vi "OCR_Seperate characters into bit arrays.vi"(7 "Color Set":T2={"BG"=255, "FG"=16711680}, 8 "Error":errorcluster, 9 "Column Type Array":T3[](array[typedef]), 11 "2D Image":u32[][](array[colorbox])) -> (0 "Error Out":errorcluster, 2 "All Good Out":bool, 3 "Char Array Out":T1[](array[typedef]))   [LabVIEW 2009]
doc: "Builds the bit character array from Image, color set, and column type array"
uses:
  Controls/Enum/ENUM_Line Letter Type.ctl
  Controls/Cluster/Cluster_Text Color Set.ctl
  Controls/String_Picture/String Char Normal.ctl
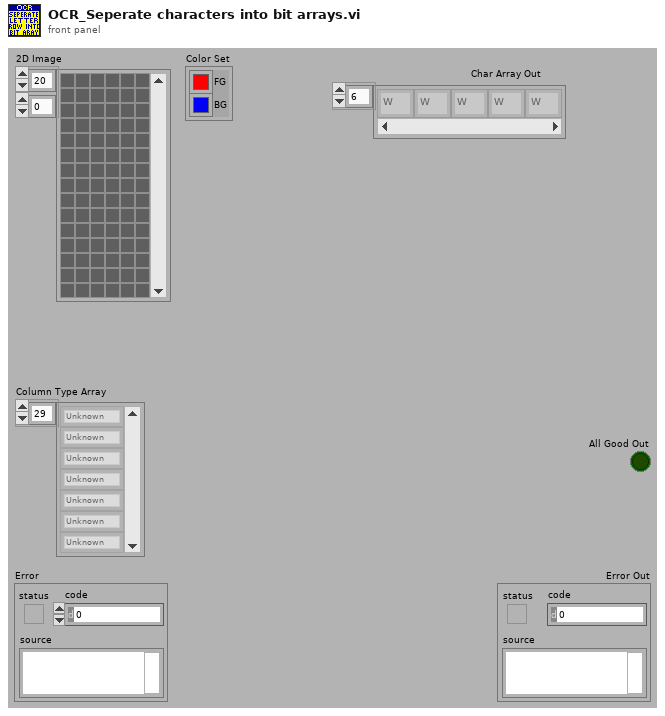
[diagram p1: front panel]
types:
  T1 = typedef "String Char Normal.ctl" = string
  T2 = typedef "Cluster_Text Color Set.ctl" = cluster{"BG":u32, "FG":u32}
  T3 = typedef "ENUM_Line Letter Type.ctl" = enum16{"Unknown", "Letter", "Seperator", "Seperator or Letter"}
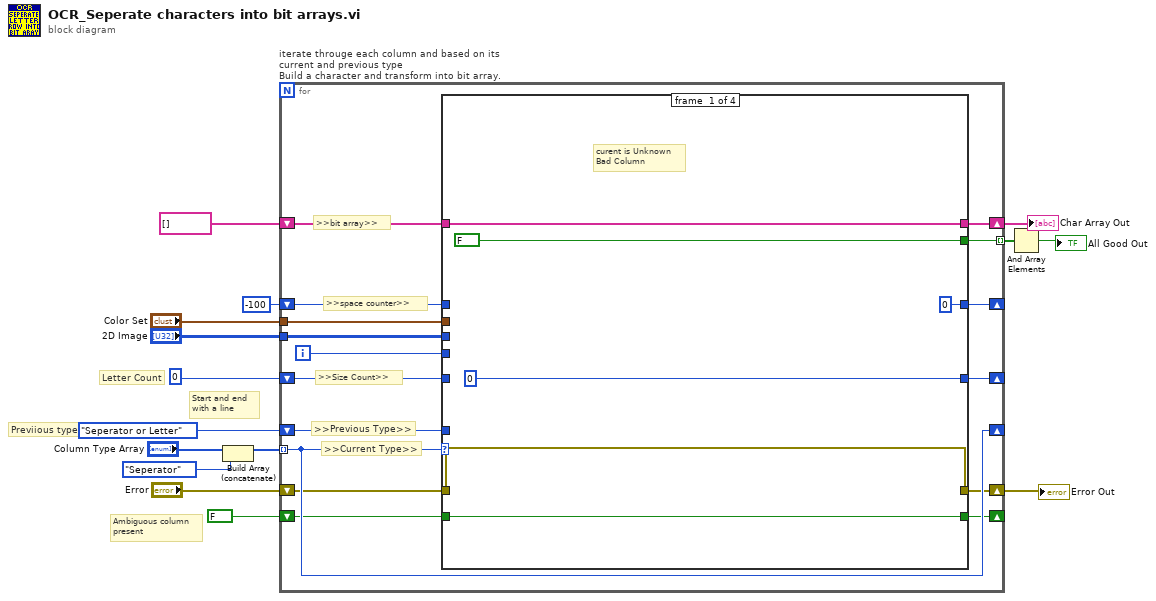
[diagram p0: block diagram]
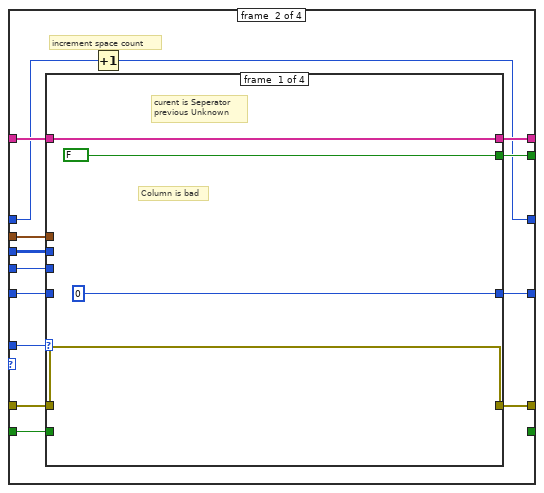
[diagram p2: hidden frame]
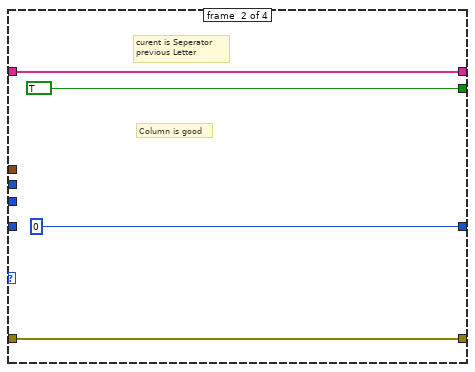
[diagram p3: hidden frame]
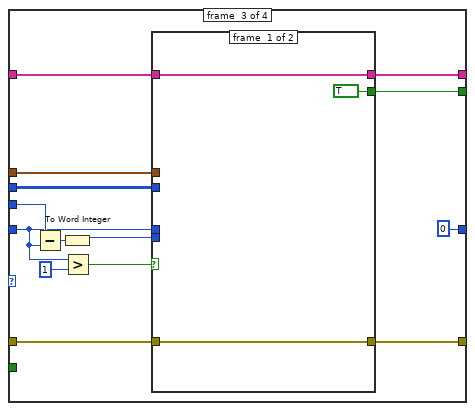
[diagram p4: hidden frame]
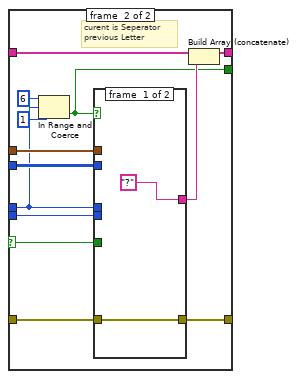
[diagram p5: hidden frame]
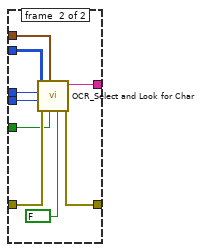
[diagram p6: hidden frame]
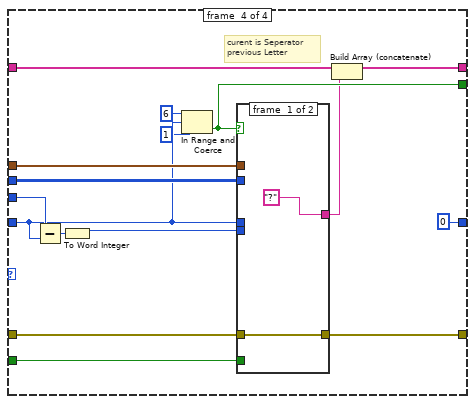
[diagram p7: hidden frame]
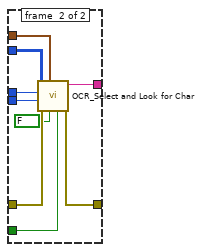
[diagram p8: hidden frame]
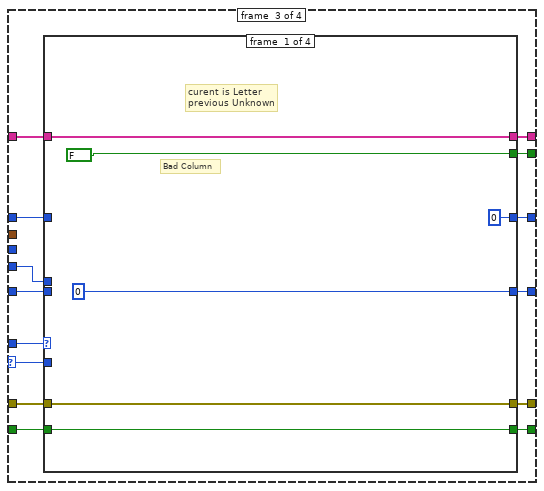
[diagram p9: hidden frame]
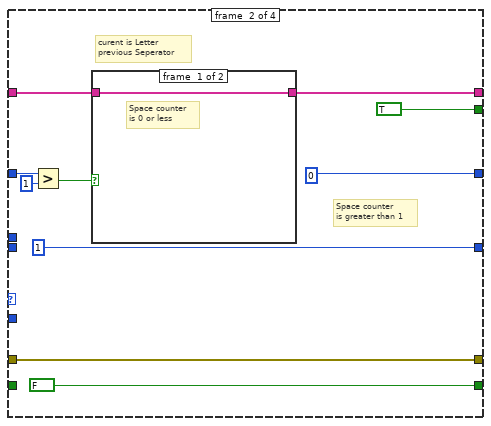
[diagram p10: hidden frame]
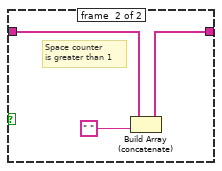
[diagram p11: hidden frame]
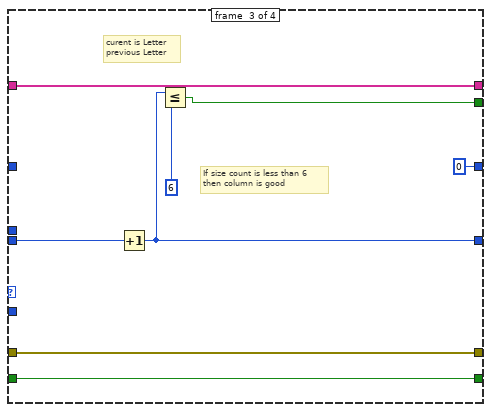
[diagram p12: hidden frame]
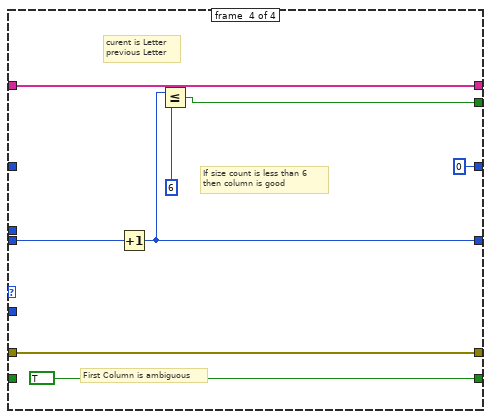
[diagram p13: hidden frame]
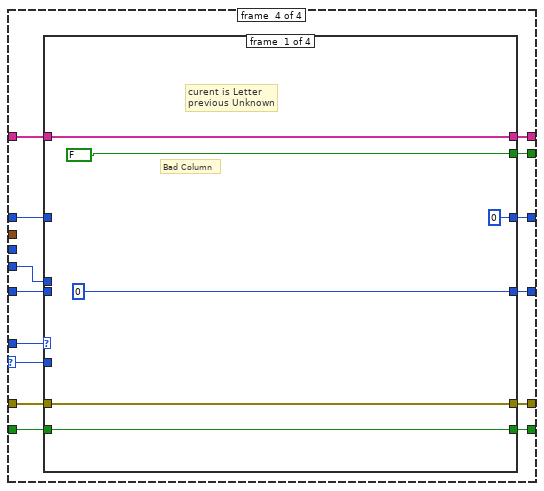
[diagram p14: hidden frame]
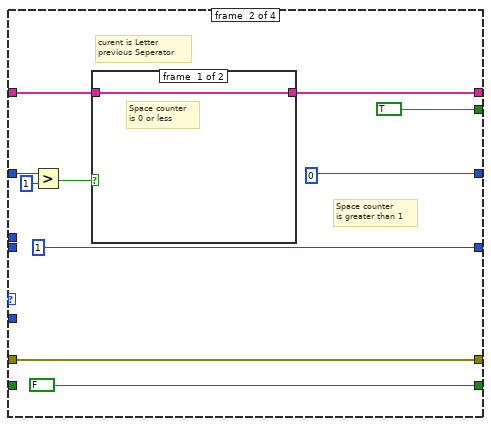
[diagram p15: hidden frame]
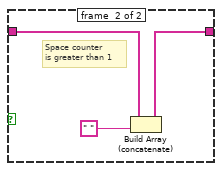
[diagram p16: hidden frame]
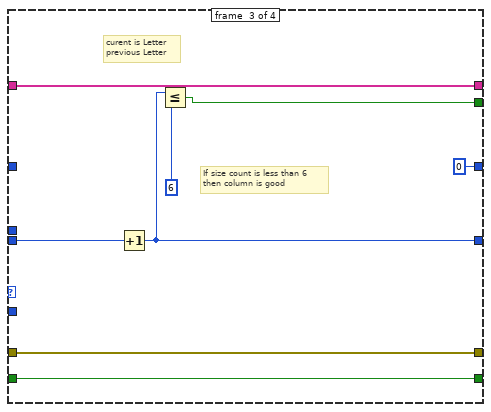
[diagram p17: hidden frame]
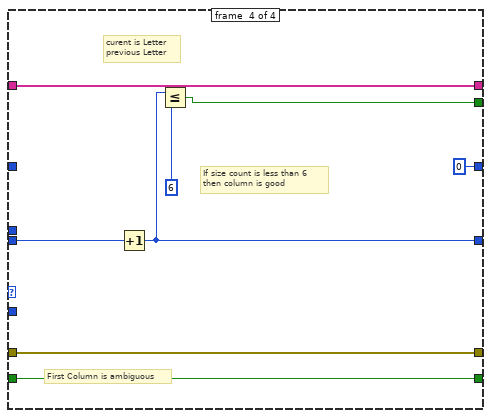
[diagram p18: hidden frame]
diagram:
  # "Ambiguous column\npresent"
  # "Start and end\nwith a line"
  # "Previious type"
  # "Letter Count"
  n1 = Build Array (concatenate)("Column Type Array", ENUM_Line_Letter_Type."Seperator" ("Type Out")) -> (w11:T3[])
  n2 = for "iterate througe each column and based on its current and previous type\nBuild a character and transform into bit array." {
    tunnel: w11 -> [w27] mode=indexing
    shift-right: [w18] -> w14
    shift-left: "Error" -> [w19]
    shift-right: [w29] -> _
    shift-left: 0 -> [w30]
    shift-right: [w27] -> _
    shift-left: ENUM_Line_Letter_Type."Seperator or Letter" ("Type Out") -> [w31]
    tunnel: "2D Image" -> [w26]
    shift-right: [w25] -> w5
    shift-left: T1[] [] ("Bit Char Array Out") -> [w24]
    tunnel: "Color Set" -> [w23]
    tunnel: [w22] -> w9 mode=indexing
    shift-right: [w20] -> _
    shift-left: -100 -> [w21]
    shift-right: [w16] -> _
    shift-left: FALSE -> [w17]
    i -> [w28]
    # ">>Size Count>>"
    # ">>Previous Type>>"
    # ">>Current Type>>"
    # ">>bit array>>"
    # ">>space counter>>"
    n3 = case shown="\"Seperator\"" w27 {
      selector: w27 -> [_ _ w132 w182]
      tunnel: w31 -> [_ w48 w138 w188]
      tunnel: w30 -> [_ w50 w140 w190]
      tunnel: [0 w51 w141 w191] -> w29
      tunnel: w28 -> [_ w49 w139 w189]
      tunnel: w26 -> [_ w47 _ _]
      tunnel: [w36 w46 w136 w186] -> w25
      tunnel: w24 -> [w36 w45 w137 w187]
      tunnel: w23 -> [_ w44 _ _]
      tunnel: [FALSE w43 w135 w185] -> w22
      tunnel: w21 -> [_ w42 w134 w184]
      tunnel: [0 w41 w133 w183] -> w20
      tunnel: w19 -> [w33 w40 w129 w179]
      tunnel: [w33 w39 w128 w178] -> w18
      tunnel: w17 -> [w32 w38 w130 w180]
      tunnel: [w32 _ w131 w181] -> w16
      frame #0 {
        # "curent is Unknown\nBad Column"
      }
      frame #1 {
        # "increment space count"
        n4 = case shown="\"Letter\"" w48 {
          tunnel: [0 0 0 0] -> w51
          tunnel: w50 -> [_ _ w62 w104]
          tunnel: w49 -> [_ _ w66 w109]
          tunnel: w47 -> [_ _ w68 w111]
          tunnel: [w54 w58 w71 w114] -> w46
          tunnel: w45 -> [w54 w58 w70 w113]
          tunnel: w44 -> [_ _ w69 w112]
          tunnel: [FALSE TRUE w63 w106] -> w43
          tunnel: w40 -> [w52 w56 w67 w110]
          tunnel: [w52 w56 w64 w107] -> w39
          tunnel: w38 -> [_ _ _ w105]
          frame #0 {
            # "curent is Seperator\nprevious Unknown"
            # "Column is bad"
          }
          frame #1 {
            # "Column is good"
            # "curent is Seperator\nprevious Letter"
          }
          frame #2 {
            n5 = Subtract(x=w66, y=w62) -> (x-y=w72:i32)
            n6 = To Word Integer(number=w72) -> (16bit integer=w65:i16)
            n7 = Greater?(x=w62, y=1) -> (0:w60:bool)
            n8 = case shown="True" w60 {
              selector: w60 -> [_ w77]
              tunnel: [w75 w89] -> w71
              tunnel: w70 -> [w75 w88]
              tunnel: w69 -> [_ w85]
              tunnel: w68 -> [_ w84]
              tunnel: w67 -> [w74 w83]
              tunnel: w62 -> [_ w82]
              tunnel: w65 -> [_ w81]
              tunnel: [w74 w80] -> w64
              tunnel: [TRUE w78] -> w63
              frame #0 {
              }
              frame #1 {
                # "curent is Seperator\nprevious Letter"
                n9 = In Range and Coerce(upper limit=6, x=w82, lower limit=1 ("y")) -> (In Range?=w78:bool)  [unwired: 1 out]
                n10 = case shown="True" w78 {
                  tunnel: w85 -> [_ w95]
                  tunnel: w84 -> [_ w96]
                  tunnel: w83 -> [w91 w100]
                  tunnel: [w91 w99] -> w80
                  tunnel: w82 -> [_ w97]
                  tunnel: w81 -> [_ w98]
                  tunnel: [T1 "?" ("Char Out") w94] -> w79
                  tunnel: w77 -> [_ w93]
                  frame #0 {
                  }
                  frame #1 {
                    n11 = call "OCR_Select and Look for Char.vi"("Ambiguous\nat Beginning"=FALSE ("Ambiguous\nat Beginning"), "Ambiguous\nat End"=w93, "Color Set"=w95, "Error"=w100, "Index"=w98, "Width"=w97, "2D Image"=w96) -> ("Error Out"=w99:errorcluster, "Char Out"=w94:T1)  [unwired: 3 in]
                  }
                }
                n12 = Build Array (concatenate)(w88, w79) -> (w89:T1[])
              }
            }
          }
          frame #3 {
            # "curent is Seperator\nprevious Letter"
            n13 = Subtract(x=w109, y=w104) -> (x-y=w115:i32)
            n14 = To Word Integer(number=w115) -> (16bit integer=w108:i16)
            n15 = In Range and Coerce(upper limit=6, x=w104, lower limit=1 ("y")) -> (In Range?=w106:bool)  [unwired: 1 out]
            n16 = case shown="True" w106 {
              tunnel: w112 -> [_ w122]
              tunnel: w111 -> [_ w123]
              tunnel: w110 -> [w118 w127]
              tunnel: [w118 w126] -> w107
              tunnel: w104 -> [_ w124]
              tunnel: w108 -> [_ w125]
              tunnel: [T1 "?" ("Char Out") w121] -> w101
              tunnel: w105 -> [_ w120]
              frame #0 {
              }
              frame #1 {
                n17 = call "OCR_Select and Look for Char.vi"("Ambiguous\nat Beginning"=w120, "Ambiguous\nat End"=FALSE ("Ambiguous\nat End"), "Color Set"=w122, "Error"=w127, "Index"=w125, "Width"=w124, "2D Image"=w123) -> ("Error Out"=w126:errorcluster, "Char Out"=w121:T1)  [unwired: 3 in]
              }
            }
            n18 = Build Array (concatenate)(w113, w101) -> (w114:T1[])
          }
        }
        n19 = Increment(x=w42) -> (x+1=w41:i32)
      }
      frame #2 {
        n20 = case shown="\"Letter\"" w138 {
          tunnel: [0 1 w167 w175] -> w141
          tunnel: w140 -> [_ _ w169 w177]
          tunnel: w139 -> [_ _ _ _]
          tunnel: w137 -> [w146 w155 w168 w176]
          tunnel: [w146 w154 w168 w176] -> w136
          tunnel: [FALSE TRUE w165 w173] -> w135
          tunnel: w134 -> [_ w152 _ _]
          tunnel: [0 0 0 0] -> w133
          tunnel: w132 -> [_ _ _ _]
          tunnel: [w143 FALSE w163 TRUE] -> w131
          tunnel: w130 -> [w143 _ w163 _]
          tunnel: w129 -> [w142 w148 w162 w171]
          tunnel: [w142 w148 w162 w171] -> w128
          frame #0 {
            # "Bad Column"
            # "curent is Letter\nprevious Unknown"
          }
          frame #1 {
            # "curent is Letter\nprevious Seperator"
            # "Space counter\nis greater than 1"
            n21 = Greater?(x=w152, y=1) -> (0:w150:bool)
            n22 = case shown="False" w150 {
              tunnel: w155 -> [w158 w161]
              tunnel: [w158 w160] -> w154
              frame #0 {
                # "Space counter\nis 0 or less"
              }
              frame #1 {
                # "Space counter\nis greater than 1"
                n23 = Build Array (concatenate)(w161, T1 " " ("Char")) -> (w160:T1[])
              }
            }
          }
          frame #2 {
            # "If size count is less than 6\nthen column is good"
            # "curent is Letter\nprevious Letter"
            n24 = Increment(x=w169) -> (x+1=w167:i32)
            n25 = Less Or Equal?(x=w167, y=6) -> (x <= y?=w165:bool)
          }
          frame #3 {
            # "First Column is ambiguous"
            # "If size count is less than 6\nthen column is good"
            # "curent is Letter\nprevious Letter"
            n26 = Increment(x=w177) -> (x+1=w175:i32)
            n27 = Less Or Equal?(x=w175, y=6) -> (x <= y?=w173:bool)
          }
        }
      }
      frame #3 {
        n28 = case shown="\"Seperator\"" w188 {
          tunnel: [0 1 w217 w225] -> w191
          tunnel: w190 -> [_ _ w219 w227]
          tunnel: w189 -> [_ _ _ _]
          tunnel: w187 -> [w196 w205 w218 w226]
          tunnel: [w196 w204 w218 w226] -> w186
          tunnel: [FALSE TRUE w215 w223] -> w185
          tunnel: w184 -> [_ w202 _ _]
          tunnel: [0 0 0 0] -> w183
          tunnel: w182 -> [_ _ _ _]
          tunnel: [w193 FALSE w213 w220] -> w181
          tunnel: w180 -> [w193 _ w213 w220]
          tunnel: w179 -> [w192 w198 w212 w221]
          tunnel: [w192 w198 w212 w221] -> w178
          frame #0 {
            # "Bad Column"
            # "curent is Letter\nprevious Unknown"
          }
          frame #1 {
            # "curent is Letter\nprevious Seperator"
            # "Space counter\nis greater than 1"
            n29 = Greater?(x=w202, y=1) -> (0:w200:bool)
            n30 = case shown="False" w200 {
              tunnel: w205 -> [w208 w211]
              tunnel: [w208 w210] -> w204
              frame #0 {
                # "Space counter\nis 0 or less"
              }
              frame #1 {
                # "Space counter\nis greater than 1"
                n31 = Build Array (concatenate)(w211, T1 " " ("Char")) -> (w210:T1[])
              }
            }
          }
          frame #2 {
            # "If size count is less than 6\nthen column is good"
            # "curent is Letter\nprevious Letter"
            n32 = Increment(x=w219) -> (x+1=w217:i32)
            n33 = Less Or Equal?(x=w217, y=6) -> (x <= y?=w215:bool)
          }
          frame #3 {
            # "First Column is ambiguous"
            # "If size count is less than 6\nthen column is good"
            # "curent is Letter\nprevious Letter"
            n34 = Increment(x=w227) -> (x+1=w225:i32)
            n35 = Less Or Equal?(x=w225, y=6) -> (x <= y?=w223:bool)
          }
        }
      }
    }
  }
  "Error Out" <- w14
  "Char Array Out" <- w5
  n36 = And Array Elements(Boolean array=w9) -> (logical AND=→"All Good Out":bool)
